vi "GVS Is Active DataView.vi"(11 "DataView Index":i32) -> (3 "bResult":bool)   [LabVIEW 2013]
uses:
  GVSNew View Global.vi
  SubVI/GVSMain Sub Window Global.vi
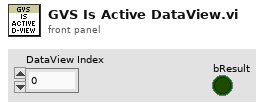
[diagram p1: front panel]
types:
  T1 = typedef "Graph Main Info Cluster.ctl" = cluster{"Selected_BarIdx":i32, "Selected_PanelIdx":i32, "Graph Main VIRef":refnum<vi>, "ToolBarClick":bool, "Spliter Ref Array":refnum<vi>[], "Panel Ref Array":refnum<vi>[], "Spliter_matrix":i32[][], "Panel_matrix":i32[][], "child_spliterIdx_matrix":i32[][], "split_pos_matrix":i32[][], "Title State":bool, "sQueueName":string, "Frame nID":i32, "Graph VIRef Array":cluster{"Graph VIRef":refnum<vi>, "Panel Idx":i32, "Frame VIRef":refnum<vi>, "Icon Ring":i32, "Graph Type":string}[], "View Type":string}
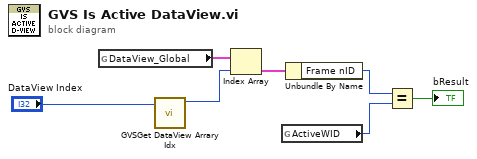
[diagram p0: block diagram]
diagram:
  n1 = global read "GVSNew View Global.vi" "DataView_Global"() -> (w7:T1[])
  n2 = call "GVSGet DataView Arrary Idx.vi"("DataView Idx In"="DataView Index") -> ("DataView Arrary Idx out"=w5:i32)  [unwired: 10 in]
  n3 = Index Array(array=w7, index=w5) -> (element=w4:T1)
  n4 = global read "GVSMain Sub Window Global.vi" "ActiveWID"() -> (w2:i32)
  n5 = Unbundle By Name(w4) -> ("Frame nID"=w3:i32)
  n6 = Equal?(x=w3, y=w2) -> (x = y?=→"bResult":bool)
